vi "PH_PowerUnit_BaseClass.PC Seq SM.vi"(0 "i ref in":refnum<vi>, 2 "SM State":string="no info", 3 "no link":bool, 5 "error in":errorcluster) -> (14 "i ref out":refnum<vi>, 19 "error out":errorcluster)   [LabVIEW 2014, in "PH_PowerUnit_BaseClass.lvlib"]
doc: "This VI writes the incoming information to own attributes and sets GUI elements."
uses:
  PH_PowerUnit_BaseClass.lvlib
  PH_Common/PH_Common.lvlib
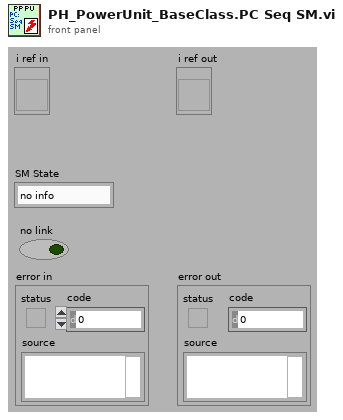
[diagram p1: front panel]
types:
  T1 = typedef "PH_PowerUnit_BaseClass.lvlib/PH_PowerUnit_BaseClass.i attribute.ctl" = cluster{"Constructor finished":bool, "PU":cluster{"In use":bool, "Service ID in use":i32, "GUI Ref":refnum<vi>}, "Enabling":cluster{"State":T2, "GUI Ref":refnum<vi>}, "Timing":cluster{"Last Shot":dbl, "Time between Shots [Sec]":dbl, "Waiting Time over?":bool, "Service ID Waiting Time":i32, "GUI Ref":refnum<vi>, "Instance":cluster{"Status":T3, "linked?":bool, "GUI Ref":refnum<vi>}}, "Sequencer":cluster{"SM State":string, "GUI Ref":refnum<vi>, "linked":bool}, "Subscribed Trendmssgs":cluster{"Tagname":string, "Status":T3, "linked?":bool, "Shot Condition":T3, "GUI Ref":refnum<vi>}[], "PP PU":T4, "Default Voltage (V)":dbl, "GUI Refs":T5, "PSDB data":cluster{"Shot Voltage [V]":dbl, "State TO SM":T6, "Write 2 early":bool}, "State TO SM":T6}
  T2 = typedef "PH_SystemInformation.lvlib/PH_SystemInformationEnabling State.ctl" = i32
  T3 = typedef "PH_StatusHandler.lvlib/PH_StatusHandler.Status.ctl" = i16
  T4 = typedef "PH_PP_Common.lvlib/PH_PP_Common.PUs.ctl" = enum16{"no Info", "PA-19mm-1", "PA-19mm-2", "PA-45mm-PILC", "PA-45mm-MAIN", "MA-PU-1", "MA-PU-2", "MA-PU-3", "MA-PU-4", "MA-PU-5", "MA-PU-6", "MA-FR", "MA-PILC", "PA-45mm-DP"}
  T5 = typedef "PH_PowerUnit_BaseClass.lvlib/PH_PowerUnit_BaseClass.GUI Refs.ctl" = cluster{"Delete Inst":refnum<vi>, "State TO SM":refnum<vi>, "State SM":refnum<vi>, "Fire":refnum<vi>}
  T6 = typedef "PH_PowerUnit_BaseClass.lvlib/PH_PowerUnit_BaseClass.SM States.ctl" = enum16{".", "Stand by", "Switch PU on", "Configure", "Set Default Voltage", "Set STANDBY", "Set READY", "Wait for Shot Cmd", "Open Dump Rods", "Open Ross Relais", "Close Ross Relais", "Switch PSU on", "Switch PSU off", "Charge", "Switch GD Channel on", "Close Dump Rods", "Rods-TO", "RR-TO", "PSU-TO", "Trigger-TO"}
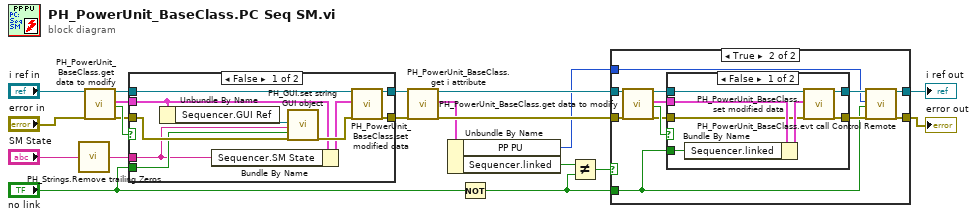
[diagram p0: block diagram]
diagram:
  n1 = call "PH_Strings.Remove trailing Zeros.vi"("Input String"="SM State") -> ("Output String"=w13:string)
  n2 = call "PH_PowerUnit_BaseClass.get data to modify.vi"("i ref in"="i ref in", "error in (no error)"="error in") -> ("i ref out"=w16:refnum<vi>, "i attribute"=w19:T1, "timed out"=w20:bool, "error out"=w18:errorcluster)  [unwired: 14 in]
  n3 = case shown="False" w20 {
    tunnel: w16 -> [w30 w32]
    tunnel: [w29 w32] -> w8
    tunnel: w18 -> [w27 w31]
    tunnel: [w28 w31] -> w10
    tunnel: w19 -> [w24 _]
    tunnel: "no link" -> [w25 _]
    tunnel: w13 -> [w21 _]
    frame False {
      n4 = Unbundle By Name(w24) -> ("Sequencer.GUI Ref"=w22:refnum<vi>)
      n5 = Bundle By Name(cluster=w24, "Sequencer.SM State"=w21) -> (w23:T1)
      n6 = call "PH_GUI.set string GUI object.vi"("GUI object Ref"=w22, "Text"=w21, "Blinking? (false)"=w25, "error in"=w27) -> ("error out"=w26:errorcluster)  [unwired: 15 in]
      n7 = call "PH_PowerUnit_BaseClass.set modified data.vi"("i ref in"=w30, "i attribute"=w23, "error in (no error)"=w26) -> ("i ref out"=w29:refnum<vi>, "error out"=w28:errorcluster)  [unwired: 15 in]
    }
    frame True {
    }
  }
  n8 = call "PH_PowerUnit_BaseClass.get i attribute.vi"("i ref in"=w8, "error in (no error)"=w10) -> ("i ref out"=w7:refnum<vi>, "i attribute"=w5:T1, "error out"=w9:errorcluster)  [unwired: 15 in]
  n9 = Unbundle By Name(w5) -> ("PP PU"=w1:T4, "Sequencer.linked"=w4:bool)
  n10 = Not(x="no link") -> (.not. x?=w3:bool)
  n11 = Not Equal?(x=w4, y=w3) -> (x != y?=w2:bool)
  n12 = case shown="True" w2 {
    tunnel: [w34 w38] -> w12
    tunnel: [w33 w39] -> w11
    tunnel: w9 -> [w33 w41]
    tunnel: w7 -> [w34 w40]
    tunnel: w3 -> [_ w37]
    tunnel: w1 -> [_ w35]
    frame False {
    }
    frame True {
      n13 = call "PH_PowerUnit_BaseClass.get data to modify.vi"("i ref in"=w40, "error in (no error)"=w41) -> ("i ref out"=w46:refnum<vi>, "i attribute"=w45:T1, "timed out"=w44:bool, "error out"=w43:errorcluster)  [unwired: 14 in]
      n14 = case shown="False" w44 {
        tunnel: w46 -> [w53 w55]
        tunnel: [w52 w55] -> w36
        tunnel: w43 -> [w47 w54]
        tunnel: [w51 w54] -> w42
        tunnel: w45 -> [w50 _]
        tunnel: w37 -> [w48 _]
        frame False {
          n15 = Bundle By Name(cluster=w50, "Sequencer.linked"=w48) -> (w49:T1)
          n16 = call "PH_PowerUnit_BaseClass.set modified data.vi"("i ref in"=w53, "i attribute"=w49, "error in (no error)"=w47) -> ("i ref out"=w52:refnum<vi>, "error out"=w51:errorcluster)  [unwired: 15 in]
        }
        frame True {
        }
      }
      n17 = call "PH_PowerUnit_BaseClass.evt call Control Remote.vi"("i ref in"=w36, "PowerUnit"=w35, "Remote controlled?"=w37, "error in (no error)"=w42) -> ("i ref out"=w38:refnum<vi>, "error out"=w39:errorcluster)  [unwired: 14 in]
    }
  }
  "error out" <- w11
  "i ref out" <- w12
